vi "freqIMU.vi"(1 "Accel DLPF Bandwidth":T2(ring), 2 "Gyro DLPF Bandwidth":T2(ring), 3 "Sample Rate Scaling":u8, 4 "SPI Config In":T1) -> (0 "SPI Config Out":T1)   [LabVIEW 2019]
uses:
  SPI/SPI Config.ctl
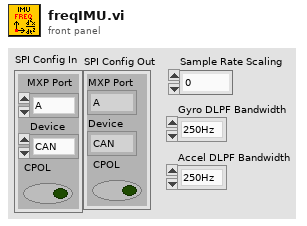
[diagram p1: front panel]
types:
  T1 = typedef "SPI Config.ctl" = cluster{"MXP Port":enum16{"A", "B"}, "Device":enum16{"CAN", "ENC", "IMU1", "IMU2"}, "CPOL":bool}
  T2 = enum16{"250Hz", "184Hz", "92Hz", "41Hz", "20Hz", "10Hz", "5Hz", "3600Hz"}
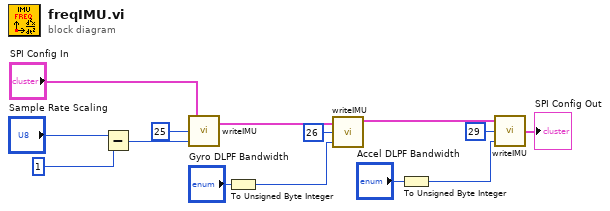
[diagram p0: block diagram]
diagram:
  n1 = Subtract(x="Sample Rate Scaling", y=u8 1) -> (x-y=w7:u8)
  n2 = call "writeIMU.vi"("Data"=w7, "Address"=u8 25, "SPI Config In"="SPI Config In") -> ("SPI Config Out"=w11:T1)
  n3 = To Unsigned Byte Integer(number="Gyro DLPF Bandwidth") -> (unsigned 8bit integer=w8:u8)
  n4 = call "writeIMU.vi"("Data"=w8, "Address"=u8 26, "SPI Config In"=w11) -> ("SPI Config Out"=w5:T1)
  n5 = To Unsigned Byte Integer(number="Accel DLPF Bandwidth") -> (unsigned 8bit integer=w2:u8)
  n6 = call "writeIMU.vi"("Data"=w2, "Address"=u8 29, "SPI Config In"=w5) -> ("SPI Config Out"=→"SPI Config Out":T1)
